vi "SEQ Obtain.vi"(8 "error in (no error)":errorcluster, 11 "Queue Name":string) -> (0 "error out":errorcluster, 3 "queue out":refnum<queue>)   [LabVIEW 2019, in "ADLINK Motion Card.lvlib"]
uses:
  ADLINK Motion Card.lvlib
  SEQ Data.ctl
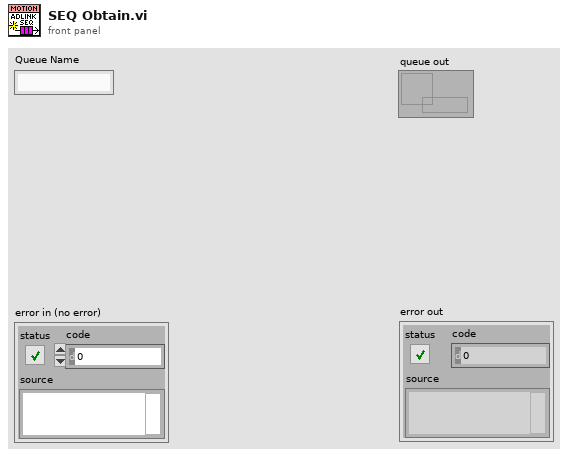
[diagram p1: front panel]
types:
  T1 = typedef "ADLINK Motion Card.lvlib/SEQ Data.ctl" = cluster{"Current Position":dbl, "Target Position":dbl, "Velocity":dbl, "Acceleration":dbl, "Arrived?":bool, "data value reference":refnum<data-value>, "VI Refnum":refnum<vi>}
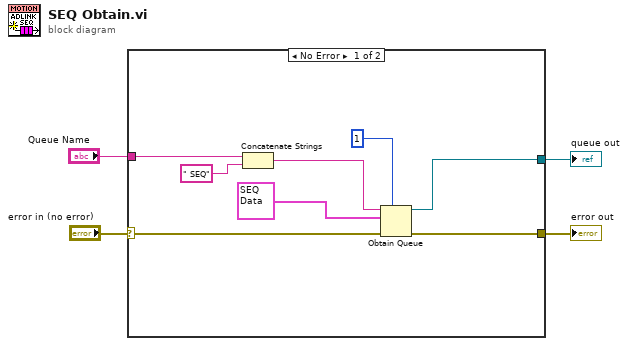
[diagram p0: block diagram]
diagram:
  n1 = case shown="No Error" "error in (no error)" {
    selector: "error in (no error)" -> [w12 w13]
    tunnel: "Queue Name" -> [w10 _]
    tunnel: [w11 w13] -> w2
    tunnel: [w5 _] -> w1
    frame No Error {
      n2 = Concatenate Strings(w10, " SEQ" ("string")) -> (w9:string)
      n3 = Obtain Queue(max queue size (-1, unlimited)=1, name (unnamed)=w9, element data type=T1 {"Current Position"=0.0, "Target Position"=0.0, "Velocity"=0.0, "Acceleration"=0.0, "Arrived?"=FALSE, "data value reference"=refnum, "VI Refnum"=refnum}, error in (no error)=w12) -> (queue out=w5:refnum<queue>, error out=w11:errorcluster)  [unwired: 1 in, 1 out]
    }
    frame Error {
    }
  }
  "error out" <- w2
  "queue out" <- w1
